vi "Regulation.vi"(6 "PID Cluster":T2={"L1 to L4 PID Cluster"={"L1 PID Gains"={"Kp"=0.005, "Kd"=0.5, "Ki"=0.0005}, "L2 PID Gains"={"Kp"=0.01, "Kd"=1.0, "Ki"=0.005}, "L3 PID Gains"={"Kp"=0.05, "Kd"=1.0, "Ki"=0.0005}, "L4 PID Gains"={"Kp"=0.1, "Kd"=0.1, "Ki"=0.0005}}, "Stage PID Cluster"={"Stage Z PID"={"Kp"=0.0005, "Kd"=0.001, "Ki"=0.0}, "Stage Y PID"={"Kp"=0.0003, "Kd"=0.01, "Ki"=0.0}, "Stage X PID"={"Kp"=0.0003, "Kd"=0.01, "Ki"=0.0}}, "OCT Z PID Gains"={"Kp"=0.0003, "Kd"=0.0001, "Ki"=0.01}}, 7 "Offset Home 2 RCM":dbl[](array[numeric])=[0.0, 0.0, 0.0, 0.0], 8 "error in":errorcluster, 9 "Engage Pt":dbl[](array[numeric])=[0.0, 0.0, 0.0, 0.0], 10 "Prev Posit Cluster":T3={"Prev L1 to L4 Posit"=[0.0, 0.0, 0.0, 0.0], "Prev Stage Posit"=[6.0, 6.0, 6.0], "Prev OCT Z Posit"=0.0}, 11 "FPGA VI Reference In":refnum<k20>) -> (0 "error out":errorcluster, 2 "Last Posit Cluster":T1={"Last L1 to L4 Posit"=[0.0, 0.0, 0.0, 0.0], "Last Stage Posit"=[6.0, 6.0, 6.0], "Last OCT Z Posit"=0.0}, 3 "FPGA VI Reference Out":refnum<k20>)   [LabVIEW 2016]
uses:
  <vilib>/Platform/TimedLoop/XDataNode/timing_clust.ctl
  <vilib>/Platform/TimedLoop/XDataNode/nitl_modes.ctl
  <vilib>/Platform/TimedLoop/XDataNode/wakeup.ctl
  Global Variables.vi
  <vilib>/platform/TimedLoop/XDataNode/XDataNode.xnode
  <vilib>/Platform/TimedLoop/XDataNode/XDNodeRunTimeDep.lvlib
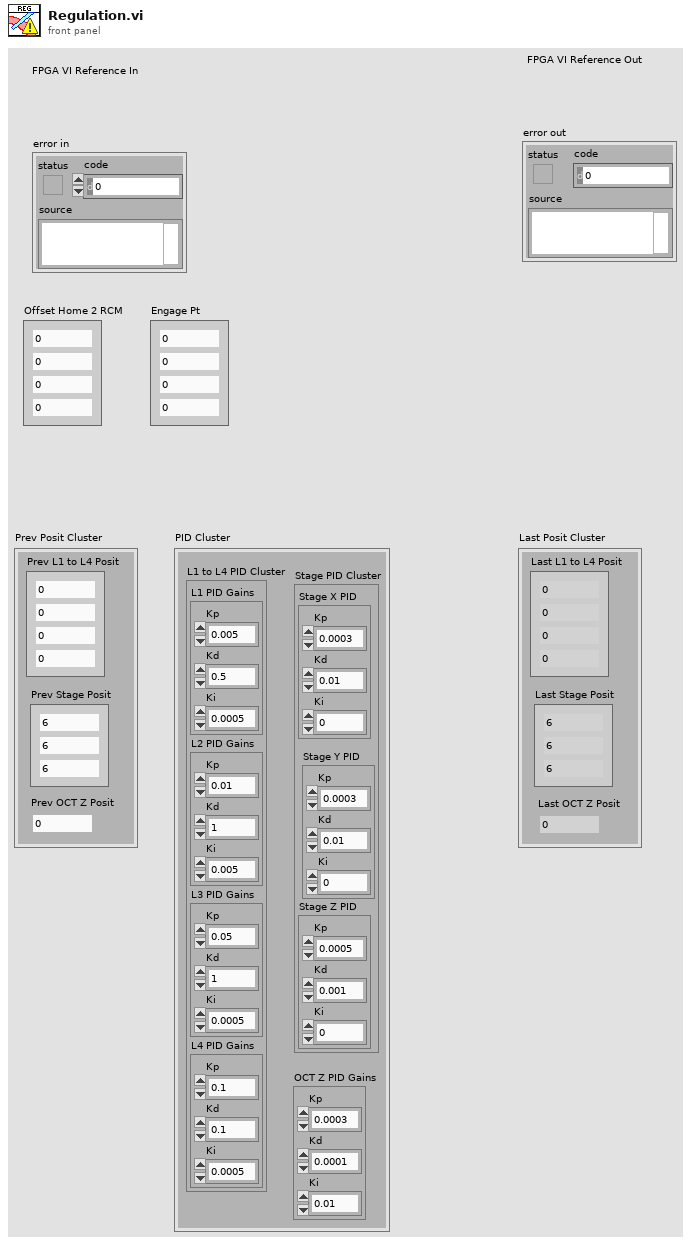
[diagram p1: front panel]
types:
  T1 = cluster{"Last L1 to L4 Posit":dbl[], "Last Stage Posit":dbl[], "Last OCT Z Posit":dbl}
  T2 = cluster{"L1 to L4 PID Cluster":cluster{"L1 PID Gains":cluster{"Kp":dbl, "Kd":dbl, "Ki":dbl}, "L2 PID Gains":cluster{"Kp":dbl, "Kd":dbl, "Ki":dbl}, "L3 PID Gains":cluster{"Kp":dbl, "Kd":dbl, "Ki":dbl}, "L4 PID Gains":cluster{"Kp":dbl, "Kd":dbl, "Ki":dbl}}, "Stage PID Cluster":cluster{"Stage Z PID":cluster{"Kp":dbl, "Kd":dbl, "Ki":dbl}, "Stage Y PID":cluster{"Kp":dbl, "Kd":dbl, "Ki":dbl}, "Stage X PID":cluster{"Kp":dbl, "Kd":dbl, "Ki":dbl}}, "OCT Z PID Gains":cluster{"Kp":dbl, "Kd":dbl, "Ki":dbl}}
  T3 = cluster{"Prev L1 to L4 Posit":dbl[], "Prev Stage Posit":dbl[], "Prev OCT Z Posit":dbl}
  T4 = cluster{"Stop Vacuum":bool, "Vacuum Force":i8, "Max Limit [mmHg]":dbl, "Slide in":i8, "Irrigation?":bool}
  T5 = typedef "XDNodeRunTimeDep.lvlib/timing_clust.ctl" = cluster{"Expected End [f-1]":u64, "Actual End [f-1]":u64, "Finished Late? [f-1]":bool, "Expected End [i-1]":u64, "Actual End [i-1]":u64, "Finished Late? [i-1]":bool, "Expected Start [i]":u64, "Actual Start [i]":u64, "Expected Start [f]":u64, "Actual Start [f]":u64, "Source Name":string, "Structure Name":string, "Period":i64, "Deadline":i64, "Offset":i64, "Start":i64, "Priority":i32, "Timeout":i32, "Mode":T6, "Wakeup Reason":T7, "Error":errorcluster, "Source Type":string, "Secondary Source Type":string, "Global End Time":u64, "Global Start Time":u64, "Frame Duration":u64, "Iteration Duration":u64, "Assigned CPU":i32, "I/O Scan Engine Mode":u32}
  T6 = typedef "XDNodeRunTimeDep.lvlib/nitl_modes.ctl" = enum32{"No Change", "Process missed periods, maintain original phase", "Discard missed periods, maintain original phase", "Process missed periods, ignore original phase", "Discard missed periods, ignore original phase"}
  T7 = typedef "XDNodeRunTimeDep.lvlib/wakeup.ctl" = enum32{"Normal", "Aborted", "Asynchronous wakeup", "Timing source error", "Timed loop error", "Timeout"}
  T8 = cluster{"Stage Z PID":cluster{"Kp":dbl, "Kd":dbl, "Ki":dbl}, "Stage Y PID":cluster{"Kp":dbl, "Kd":dbl, "Ki":dbl}, "Stage X PID":cluster{"Kp":dbl, "Kd":dbl, "Ki":dbl}}
  T9 = cluster{"L1 PID Gains":cluster{"Kp":dbl, "Kd":dbl, "Ki":dbl}, "L2 PID Gains":cluster{"Kp":dbl, "Kd":dbl, "Ki":dbl}, "L3 PID Gains":cluster{"Kp":dbl, "Kd":dbl, "Ki":dbl}, "L4 PID Gains":cluster{"Kp":dbl, "Kd":dbl, "Ki":dbl}}
  T10 = cluster{"Accurus button":bool[], "Accurus engaged?":bool, "Vacuum Force":i32, "Accurus Ch. A Vout":dbl, "Accurus Ch. B Vout":dbl, "Irrigation engaged?":bool}
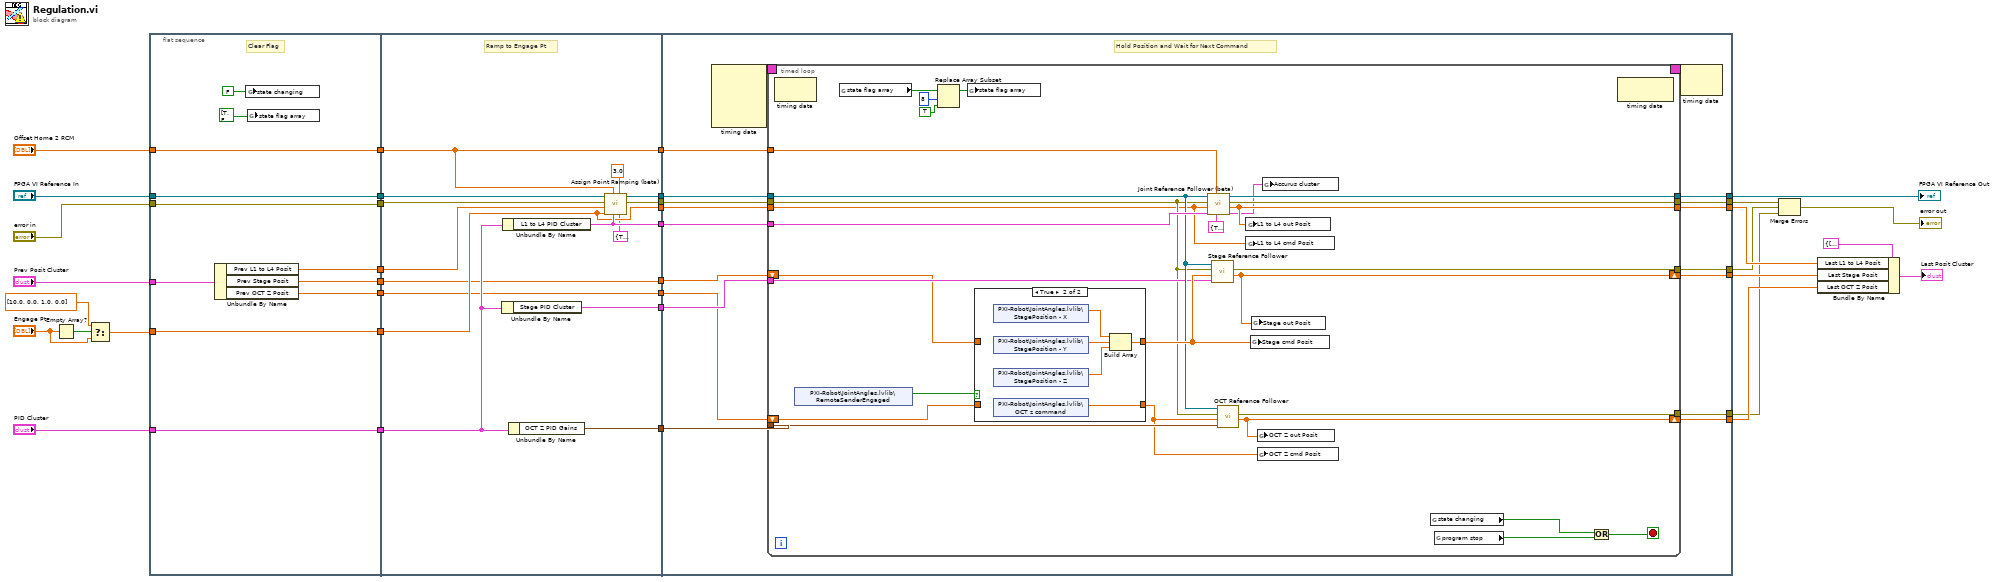
[diagram p0: block diagram]
diagram:
  n1 = Empty Array?(array="Engage Pt") -> (empty?=w28:bool)
  n2 = Select(t=dbl[] [10.0, 0.0, 1.0, 0.0] ("First Trk Pt 2"), s=w28, f="Engage Pt") -> (s? t:f=w25:dbl[])
  n3 = flat-sequence {
    tunnel: [w45] -> w36
    tunnel: "FPGA VI Reference In" -> [w45]
    tunnel: "error in" -> [w44]
    tunnel: [w44] -> w35
    tunnel: [w38] -> w34
    tunnel: "PID Cluster" -> [w42]
    tunnel: "Offset Home 2 RCM" -> [w43]
    tunnel: [w43] -> w32
    tunnel: [w37] -> w30
    tunnel: w25 -> [w37]
    tunnel: [w42] -> w18
    tunnel: "Prev Posit Cluster" -> [w41]
    tunnel: [w40] -> w4
    tunnel: [w39] -> w1
    tunnel: w36 -> [w62]
    tunnel: w35 -> [w61]
    tunnel: w34 -> [w59]
    tunnel: w32 -> [w56]
    tunnel: w30 -> [w51]
    tunnel: [w58] -> w29
    tunnel: [w51] -> w24
    tunnel: [w57] -> w23
    tunnel: [w56] -> w22
    tunnel: [w55] -> w21
    tunnel: w18 -> [w53]
    tunnel: [w54] -> w17
    tunnel: [w52] -> w16
    tunnel: w4 -> [w50]
    tunnel: [w50] -> w3
    tunnel: [w49] -> w2
    tunnel: w1 -> [w49]
    tunnel: [w74] -> w12
    tunnel: [w73] -> w7
    tunnel: w29 -> [w77]
    tunnel: w24 -> [w76]
    tunnel: w23 -> [w78]
    tunnel: w22 -> [w65]
    tunnel: w21 -> [w75]
    tunnel: [w72] -> w19
    tunnel: [w71] -> w20
    tunnel: w17 -> [w70]
    tunnel: w16 -> [w69]
    tunnel: [w68] -> w13
    tunnel: [w67] -> w6
    tunnel: [w66] -> w5
    tunnel: w3 -> [w64]
    tunnel: w2 -> [w63]
    frame #0 {
      # "Clear Flag"
      n4 = Unbundle By Name(w41) -> ("Prev L1 to L4 Posit"=w38:dbl[], "Prev Stage Posit"=w40:dbl[], "Prev OCT Z Posit"=w39:dbl)
      n5 = global write "Global Variables.vi" "state changing"(FALSE ("state changing")) -> ()
      n6 = global write "Global Variables.vi" "state flag array"(bool[] [TRUE, FALSE, FALSE, FALSE, FALSE, FALSE, FALSE, FALSE, FALSE] ("state flag array")) -> ()
    }
    frame #1 {
      # "Ramp to Engage Pt"
      n7 = Unbundle By Name(w53) -> ("Stage PID Cluster"=w54:T8)
      n8 = Unbundle By Name(w53) -> ("L1 to L4 PID Cluster"=w55:T9)
      n9 = Unbundle By Name(w53) -> ("OCT Z PID Gains"=w52:cluster{"Kp":dbl, "Kd":dbl, "Ki":dbl})
      n10 = call "Assign Point Ramping (beta).vi"("Accurus Ctrl Cluster"=T4 {"Stop Vacuum"=TRUE, "Vacuum Force"=0, "Max Limit [mmHg]"=600.0, "Slide in"=0, "Irrigation?"=TRUE}, "Ramp Time [sec]"=3.0, "L1 to L4 PID Cluster"=w55, "Offset Home2RCM"=w56, "Destination Posit Array [mm]"=w51, "Previous Posit Array"=w59, "error in"=w61, "FPGA VI Reference In"=w62) -> ("error out"=w58:errorcluster, "FPGA VI Reference Out"=w57:refnum<k20>)  [unwired: 1 in, 1 out]
    }
    frame #2 {
      # "Hold Position and Wait for Next Command"
      n11 = node-c288() -> (w80:T5)  [unwired: 4 in]
      n12 = timed-loop {
        timing: w80 -> [_]
        timing-out: [_] -> w79
        tunnel: w78 -> [w97]
        tunnel: w77 -> [w89]
        tunnel: w65 -> [w103]
        tunnel: w76 -> [w83]
        tunnel: w75 -> [w102]
        tunnel: [w101] -> w74
        tunnel: [w100] -> w73
        tunnel: [w95] -> w72
        tunnel: w70 -> [w94]
        tunnel: w69 -> [w93]
        tunnel: [w88] -> w67
        tunnel: [w87] -> w66
        shift-right: [w98] -> w71
        shift-left: w64 -> [w85]
        shift-right: [w92] -> w68
        shift-left: w63 -> [w84]
        stop <- w90 stop-if-true
        n13 = node-c288() -> ()  [unwired: 1 in, 1 out]
        n14 = shared-variable "PXI-Robot\\JointAngles.lvlib\\RemoteSenderEngaged"() -> (w86:bool)  [unwired: 1 in, 1 out]
        n15 = global read "Global Variables.vi" "state flag array"() -> (w107:bool[])
        n16 = Replace Array Subset(array=w107, new element=TRUE ("new element/subarray"), index=8) -> (w106:bool[])
        n17 = global write "Global Variables.vi" "state flag array"(w106) -> ()
        n18 = case shown="True" w86 {
          tunnel: [w110 w112] -> w99
          tunnel: [w109 w111] -> w91
          tunnel: w85 -> [w110 _]
          tunnel: w84 -> [w109 _]
          frame False {
            # "Hold Position if not Engaged"
          }
          frame True {
            n19 = shared-variable "PXI-Robot\\JointAngles.lvlib\\StagePosition - X"() -> (w115:dbl)  [unwired: 1 in, 1 out]
            n20 = shared-variable "PXI-Robot\\JointAngles.lvlib\\StagePosition - Y"() -> (w114:dbl)  [unwired: 1 in, 1 out]
            n21 = shared-variable "PXI-Robot\\JointAngles.lvlib\\StagePosition - Z"() -> (w113:dbl)  [unwired: 1 in, 1 out]
            n22 = shared-variable "PXI-Robot\\JointAngles.lvlib\\OCT z command"() -> (w111:dbl)  [unwired: 1 in, 1 out]
            n23 = Build Array(w115, w114, w113) -> (w112:dbl[])
          }
        }
        n24 = call "Joint Reference Follower (beta).vi"("Accurus Ctrl Cluster"=T4 {"Stop Vacuum"=TRUE, "Vacuum Force"=0, "Max Limit [mmHg]"=600.0, "Slide in"=0, "Irrigation?"=TRUE}, "Offset Home2RCM [deg/mm]"=w103, "PID Ctrl Cluster"=w102, "Ref Array [deg/mm]"=w83, "error in"=w89, "FPGA VI Reference In"=w97) -> ("Accurus Output Cluster"=w81:T10, "Output Posit Array [deg/mm]"=w95:dbl[], "error out"=w100:errorcluster, "FPGA VI Reference Out"=w101:refnum<k20>)  [unwired: 2 in]
        n25 = call "Stage Reference Follower.vi"("Stage PID Cluster"=w94, "Stage cmd Posit [mm]"=w99, "error in"=w89, "FPGA VI Reference In"=w97) -> ("Stage out Posit [mm]"=w98:dbl[], "error out"=w88:errorcluster)  [unwired: 5 in, 1 out]
        n26 = call "OCT Reference Follower.vi"("OCT Z PID Gains"=w93, "OCT  Z cmd Posit [mm]"=w91, "error in"=w89, "FPGA VI Reference In"=w97) -> ("OCT  Z out Posit [mm]"=w92:dbl, "error out"=w87:errorcluster)  [unwired: 5 in, 1 out]
        n27 = global write "Global Variables.vi" "L1 to L4 out Posit"(w95) -> ()
        n28 = global write "Global Variables.vi" "L1 to L4 cmd Posit"(w83) -> ()
        n29 = global write "Global Variables.vi" "Stage cmd Posit"(w99) -> ()
        n30 = global write "Global Variables.vi" "Stage out Posit"(w98) -> ()
        n31 = global write "Global Variables.vi" "OCT Z out Posit"(w92) -> ()
        n32 = global write "Global Variables.vi" "OCT Z cmd Posit"(w91) -> ()
        n33 = global write "Global Variables.vi" "Accurus cluster"(w81) -> ()
        n34 = global read "Global Variables.vi" "state changing"() -> (w108:bool)
        n35 = global read "Global Variables.vi" "program stop"() -> (w96:bool)
        n36 = Or(x=w108, y=w96) -> (x .or. y?=w90:bool)
        n37 = node-c288() -> ()  [unwired: 1 in, 1 out]
      }
      n38 = node-c288(w79) -> ()  [unwired: 1 out]
    }
  }
  n39 = Merge Errors(w7, w6, w5) -> (→"error out":errorcluster)
  n40 = Bundle By Name(cluster=T1 {"Last L1 to L4 Posit"=[0.0, 0.0, 0.0, 0.0], "Last Stage Posit"=[6.0, 6.0, 6.0], "Last OCT Z Posit"=0.0} ("Last Posit Cluster 2"), "Last L1 to L4 Posit"=w19, "Last Stage Posit"=w20, "Last OCT Z Posit"=w13) -> (→"Last Posit Cluster":T1)
  "FPGA VI Reference Out" <- w12
